vi "RGBtoXYZ.vi"(1 "RGB":dbl[](array[numeric]), 2 "Illuminants":T1, 3 "Selected RGB":string(combo)) -> (0 "XYZ":dbl[](array[numeric]))   [LabVIEW 2013]
uses:
  <vilib>/Analysis/baseanly.llb/A x Vector.vi
  <vilib>/Analysis/NI_AALBase.lvlib
panel:
  out "M":dbl[][](array[numeric])
  out "gamma":dbl
  out "RGBStandards":string[][](array[string])
  out "RGBStandardRows":i32
  out "RGBMatrix":dbl[][](array[numeric])
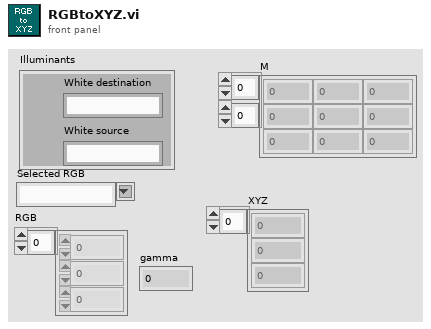
[diagram p1: front panel]
types:
  T1 = cluster{"White destination":string, "White source":string}
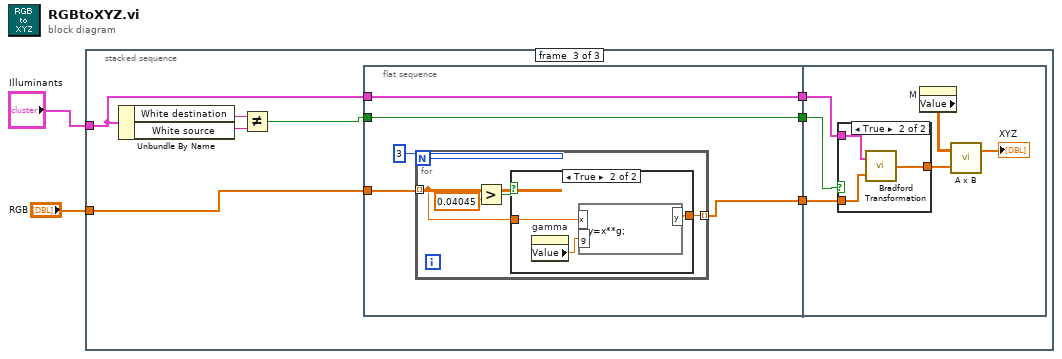
[diagram p0: block diagram]
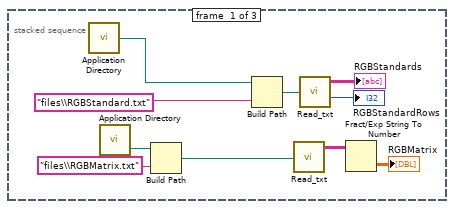
[diagram p2: hidden frame]
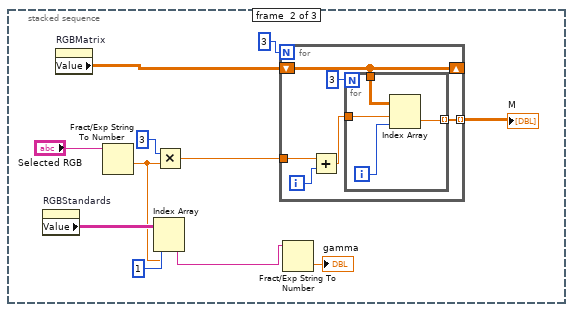
[diagram p3: hidden frame]
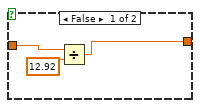
[diagram p4: hidden frame]
diagram:
  n1 = stacked-sequence {
    tunnel: "RGB" -> [_ _ w41]
    tunnel: "Illuminants" -> [_ _ w40]
    frame #0 {
      n2 = call <vilib>:"Application Directory.vi"() -> ("Application Directory"=w4:path)
      n3 = call <vilib>:"Application Directory.vi"() -> ("Application Directory"=w3:path)
      n4 = Build Path(base path=w3, name or relative path="files\\RGBMatrix.txt") -> (appended path=w7:path)
      n5 = Build Path(base path=w4, name or relative path="files\\RGBStandard.txt") -> (appended path=w5:path)
      n6 = call "Read_txt.vi"("file path (dialog if empty)"=w7) -> ("Elements"=w9:string[][])  [unwired: 2 out]
      n7 = call "Read_txt.vi"("file path (dialog if empty)"=w5) -> ("Elements"=→"RGBStandards":string[][], "Rows"=→"RGBStandardRows":i32)  [unwired: 1 out]
      n8 = Fract/Exp String To Number(string=w9) -> (number=→"RGBMatrix":dbl[][])  [unwired: 3 in, 1 out]
    }
    frame #1 {
      n9 = property on="RGBStandards" class="Arr (strict)"() -> ("Value"=w18:string[][])  [unwired: 2 in, 2 out]
      n10 = property on="RGBMatrix" class="Arr (strict)"() -> ("Value"=w20:dbl[][])  [unwired: 2 in, 2 out]
      n11 = Fract/Exp String To Number(string="Selected RGB") -> (number=w16:dbl)  [unwired: 3 in, 1 out]
      n12 = Index Array(array=w18, index (row)=w16, index (col)=1 ("disabled index (col)")) -> (element=w15:string)
      n13 = Multiply(x=3, y=w16) -> (x*y=w21:dbl)
      n14 = for {
        N: 3 -> [_]
        shift-right: [w28] -> _
        shift-left: w20 -> [w28]
        tunnel: w21 -> [w27]
        tunnel: [w24] -> w13 mode=indexing
        i -> [w26]
        n15 = Add(x=w27, y=w26) -> (x+y=w25:dbl)
        n16 = for {
          N: 3 -> [_]
          tunnel: w28 -> [w33]
          tunnel: w25 -> [w32]
          tunnel: [w31] -> w24 mode=indexing
          i -> [w30]
          n17 = Index Array(array=w33, index (row)=w32, index (col)=w30) -> (element=w31:dbl)
        }
      }
      "M" <- w13
      n18 = Fract/Exp String To Number(string=w15) -> (number=→"gamma":dbl)  [unwired: 3 in, 1 out]
    }
    frame #2 {
      n19 = Unbundle By Name(w40) -> ("White destination"=w38:string, "White source"=w39:string)
      n20 = Not Equal?(x=w38, y=w39) -> (x != y?=w37:bool)
      n21 = flat-sequence {
        tunnel: w37 -> [w43]
        tunnel: w41 -> [w45]
        tunnel: w40 -> [w42]
        tunnel: [w44] -> w36
        tunnel: [w43] -> w35
        tunnel: [w42] -> w34
        tunnel: w36 -> [w59]
        tunnel: w35 -> [w58]
        tunnel: w34 -> [w57]
        frame #0 {
          n22 = for {
            N: 3 -> [_]
            tunnel: w45 -> [w49] mode=indexing
            tunnel: [w50] -> w44 mode=indexing
            n23 = Greater?(x=w49, y=0.04045) -> (0:w47:bool)
            n24 = case shown="True" w47 {
              tunnel: [w51 w55] -> w50
              tunnel: w49 -> [w53 w56]
              frame False {
                n25 = Divide(x=w53, y=12.92) -> (x/y=w51:dbl)
              }
              frame True {
                n26 = property on="gamma" class="DigNum (strict)"() -> ("Value"=w54:dbl)  [unwired: 2 in, 2 out]
                n27 = formula code="y=x**g;"("x"=w56, "g"=w54) -> ("y"=w55:dbl)
              }
            }
          }
        }
        frame #1 {
          n28 = case shown="True" w58 {
            tunnel: w59 -> [w63 w66]
            tunnel: w57 -> [_ w65]
            tunnel: [w63 w64] -> w60
            frame False {
            }
            frame True {
              n29 = call "Bradford Transformation.vi"("XYZs"=w66, "Illuminants"=w65) -> ("XYZd"=w64:dbl[])
            }
          }
          n30 = property on="M" class="Arr (strict)"() -> ("Value"=w62:dbl[][])  [unwired: 2 in, 2 out]
          n31 = call-poly <vilib>:"A x B.vi"("Vector"=w60, "A"=w62) -> ("A x Vector"=→"XYZ":dbl[])  [unwired: 1 out]
        }
      }
    }
  }
